vi "Set all LED powers.vi"(8 "error in":errorcluster, 9 "LED Power (%)":dbl(slide) min=0.0 max=120.0 step=1.0 scale=0.0..100.0 scale format="%.1f", 11 "LED handle in":refnum<visa-resource-name>) -> (0 "error out":errorcluster {"code" format="%.0x"}, 3 "LED handle out":refnum<visa-resource-name> caption="instrument handle out")   [LabVIEW 2017]
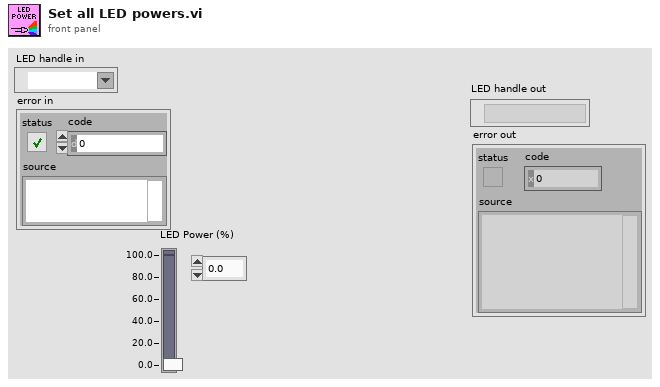
[diagram p1: front panel]
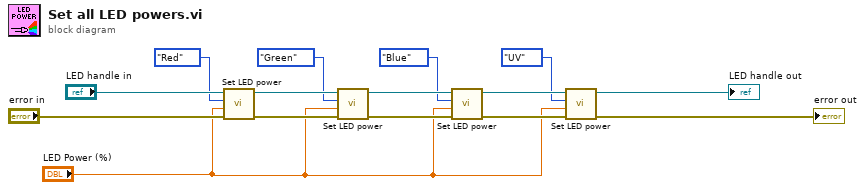
[diagram p0: block diagram]
diagram:
  n1 = call "Set LED power.vi"("error in"="error in", "LED Power (%)"="LED Power (%)", "LED"=enum8{"Red", "UV", "Green", "Blue"}."Red", "LED handle in"="LED handle in") -> ("error out"=w10:errorcluster, "LED handle out"=w9:refnum<visa-resource-name>)  [unwired: 6 in]
  n2 = call "Set LED power.vi"("error in"=w10, "LED Power (%)"="LED Power (%)", "LED"=enum8{"Red", "UV", "Green", "Blue"}."Green", "LED handle in"=w9) -> ("error out"=w11:errorcluster, "LED handle out"=w8:refnum<visa-resource-name>)  [unwired: 6 in]
  n3 = call "Set LED power.vi"("error in"=w11, "LED Power (%)"="LED Power (%)", "LED"=enum8{"Red", "UV", "Green", "Blue"}."Blue", "LED handle in"=w8) -> ("error out"=w6:errorcluster, "LED handle out"=w7:refnum<visa-resource-name>)  [unwired: 6 in]
  n4 = call "Set LED power.vi"("error in"=w6, "LED Power (%)"="LED Power (%)", "LED"=enum8{"Red", "UV", "Green", "Blue"}."UV", "LED handle in"=w7) -> ("error out"=→"error out":errorcluster, "LED handle out"=→"LED handle out":refnum<visa-resource-name>)  [unwired: 6 in]
